vi "Test-KH_CDC_Scale.vi"(11 "r":dbl) -> (3 "2byte":dbl)   [LabVIEW 2015]
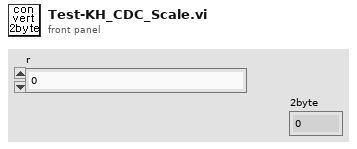
[diagram p1: front panel]
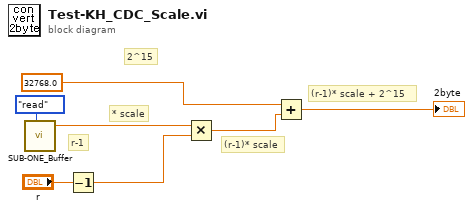
[diagram p0: block diagram]
diagram:
  # "(r-1)* scale + 2^15"
  # "(r-1)* scale"
  # "* scale"
  # "r-1"
  # "2^15"
  n1 = call "SUB-ONE_Buffer.vi"("mode"=enum16{"write", "read"}."read") -> ("OUT"=w1:dbl)  [unwired: 10 in]
  n2 = Decrement(x="r") -> (x-1=w7:dbl)
  n3 = Multiply(x=w1, y=w7) -> (x*y=w6:dbl)
  n4 = Add(x=32768.0, y=w6) -> (x+y=→"2byte":dbl)
